vi "Create new Log files.vi"(11 "Log folder":path=path "C:/HFEPR_logs") -> (0 "error out":errorcluster, 1 "dup path":path, 2 "tmp logfile out":refnum<file>, 3 "event logfile out":refnum<file>)   [LabVIEW 2022 SP3]
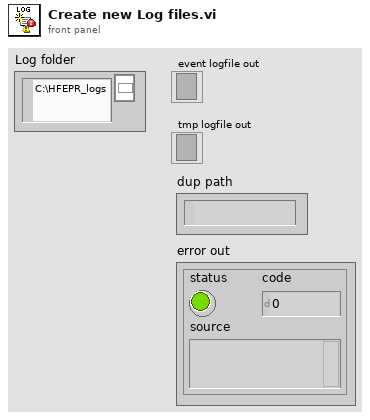
[diagram p1: front panel]
types:
  T1 = enum16{"open", "replace", "create", "open or create", "replace or create", "replace or create with confirmation"}
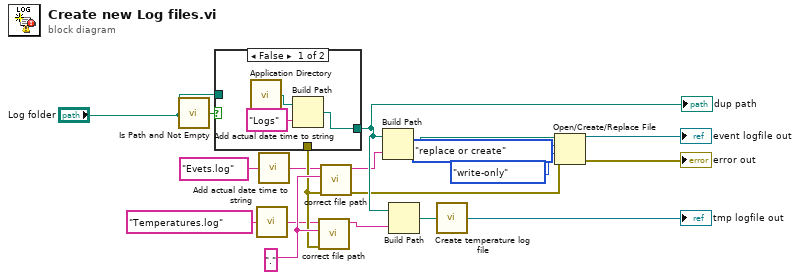
[diagram p0: block diagram]
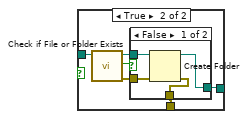
[diagram p2: hidden frame]
diagram:
  w17 = "."
  n1 = call <vilib>:"Is Path and Not Empty.vi"("path"="Log folder") -> ("Is Path and Not Empty?"=w5:bool)  [unwired: 4 in]
  n2 = case shown="False" w5 {
    tunnel: [w21 w26] -> w19
    tunnel: "Log folder" -> [_ w25]
    tunnel: [_ w23] -> w14
    frame False {
      n3 = call <vilib>:"Application Directory.vi"() -> ("Application Directory"=w22:path)
      n4 = Build Path(base path=w22, name or relative path="Logs") -> (appended path=w21:path)
    }
    frame True {
      n5 = call <vilib>:"Check if File or Folder Exists.vi"("path"=w25) -> ("error out"=w24:errorcluster, "file or folder exists?"=w27:bool, "dup path"=w28:path)  [unwired: 8 in]
      n6 = case shown="False" w27 {
        tunnel: w28 -> [w32 w34]
        tunnel: [w31 w34] -> w26
        tunnel: w24 -> [w30 w33]
        tunnel: [w29 w33] -> w23
        frame False {
          n7 = Create Folder(path (use dialog)=w32, error in=w30) -> (created path=w31:path, error out=w29:errorcluster)  [unwired: 1 in, 1 out]
        }
        frame True {
        }
      }
    }
  }
  "dup path" <- w19
  n8 = call "Add actual date time to string.vi"("String in"="Temperatures.log" ("name or relative path")) -> ("String out"=w13:string)  [unwired: 4 in]
  n9 = call "Add actual date time to string.vi"("String in"="Evets.log" ("name or relative path")) -> ("String out"=w7:string)  [unwired: 4 in]
  n10 = call "correct file path.vi"("error in (no error)"=w14, "replacement (-)"=w17, "input path"=w13) -> ("corrected path"=w15:string)  [unwired: 7 in, 1 out]
  n11 = call "correct file path.vi"("error in (no error)"=w14, "replacement (-)"=w17, "input path"=w7) -> ("error out"=w10:errorcluster, "corrected path"=w9:string)  [unwired: 7 in]
  n12 = Build Path(base path=w19, name or relative path=w9) -> (appended path=w18:path)
  n13 = Build Path(base path=w19, name or relative path=w15) -> (appended path=w16:path)
  n14 = call "Create temperature log file.vi"("path in"=w16) -> ("refnum out"=→"tmp logfile out":refnum<file>)  [unwired: 3 in, 1 out]
  n15 = Open/Create/Replace File(file path (use dialog)=w18, error in=w10, operation (0:open)=T1."replace or create", access (0:read/write)=enum16{"read/write", "read-only", "write-only"}."write-only") -> (refnum out=→"event logfile out":refnum<file>, error out=→"error out":errorcluster)  [unwired: 2 in, 1 out]
